vi "231215_Spectrometer_Example_2.0.vi"() -> ()   [LabVIEW 2026]
uses:
  Utils/Status_Ctrl.ctl
  Ocean Optics 2000 4000/Ocean Optics 2000 4000.lvlib
panel:
  in  "Tab Control 2":T1(tab)
  in  "Normalize?":bool
  in  "Source":u16(ring) items=["---", "Source 1", "Source 2", "Source 3"]
  out "Source graph":cluster{dbl[], dbl[]}[](graph)
  in  "SAVE":bool
  in  "Type of measurement":u16(ring)=2 items=["---", "Background noise", "Source without filter", "Source after the filter"]
  out "Source graph 2":cluster{dbl[], dbl[]}[](graph)
  out "Transmission_graph":cluster{dbl[], dbl[]}(graph)
  in  "File Path":path
  in  "File name (wo extension)":string
  in  "Type of curve to save":u16(ring)=2 items=["Save the transmission spectrum", "Save the source spectrum"]
  in  "Filter cluster":T2={"Type of filter"=enum."---", "Centered wavelength (nm)"=0.0, "Transmission band (nm)"=1.0, "Transmission (%)"=0.0} {"Transmission (%)" min=0.0 max=100.0 step=1.0; "Transmission band (nm)" min=1.0 step=1.0}
  out "Filter name":string
  out "Filter_Graph":cluster{dbl[], dbl[]}[](graph)
  out "Wavelength_Size":i32=3648
  in  "Tab Control":enum32{"Spectrometer", "Tools"}(tab)
  in  "Wavelength / Intensity limits":u16[][](array[numeric])=[[400, 0], [750, 2000]]
  in  "Intensity autoscale?":bool=TRUE
  in  "Averages":u8=1 min=1
  out "CurrentSpectrum":cluster{dbl[], dbl[]}(graph)
  out "Saturated!":bool
  in  "Status":T3=enum."Exit"
  in  "Integration time (ms)":u16=100 min=1
  out "error out":errorcluster
  # "Programmed by Sébastien Mailfert"
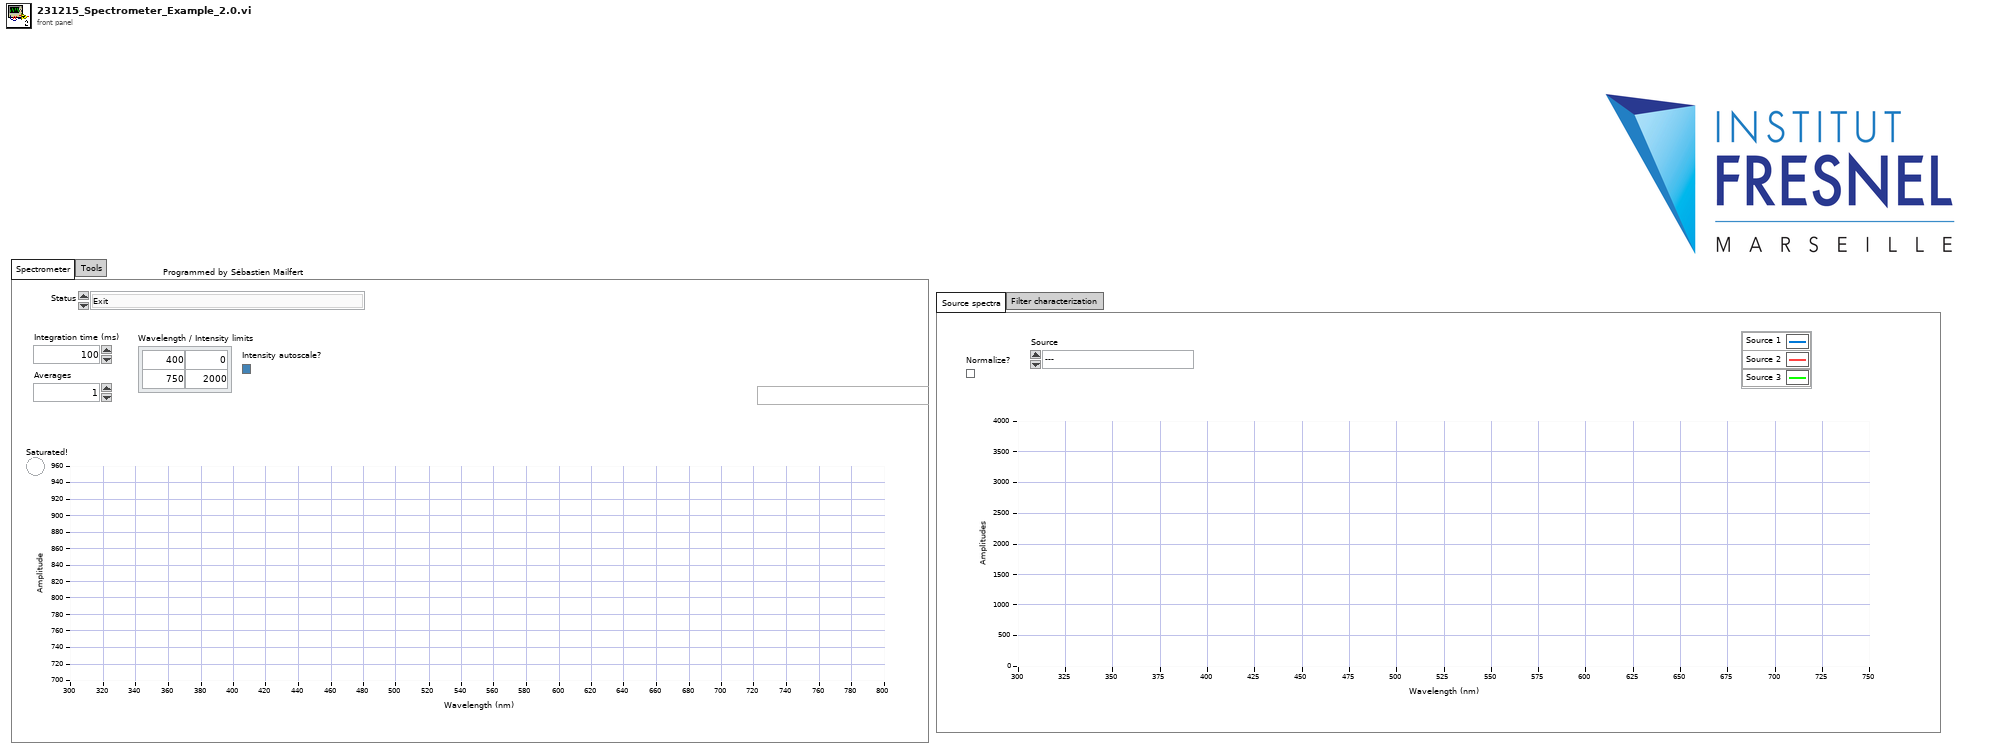
[diagram p1: front panel]
types:
  T1 = enum32{"Source spectra", "Filter characterization"}
  T2 = cluster{"Type of filter":enum16{"---", "Bandpass", "Longpass", "Shortpass"}, "Centered wavelength (nm)":dbl, "Transmission band (nm)":dbl, "Transmission (%)":dbl}
  T3 = typedef "Status_Ctrl.ctl" = enum16{"Init", "Live", "Exit"}
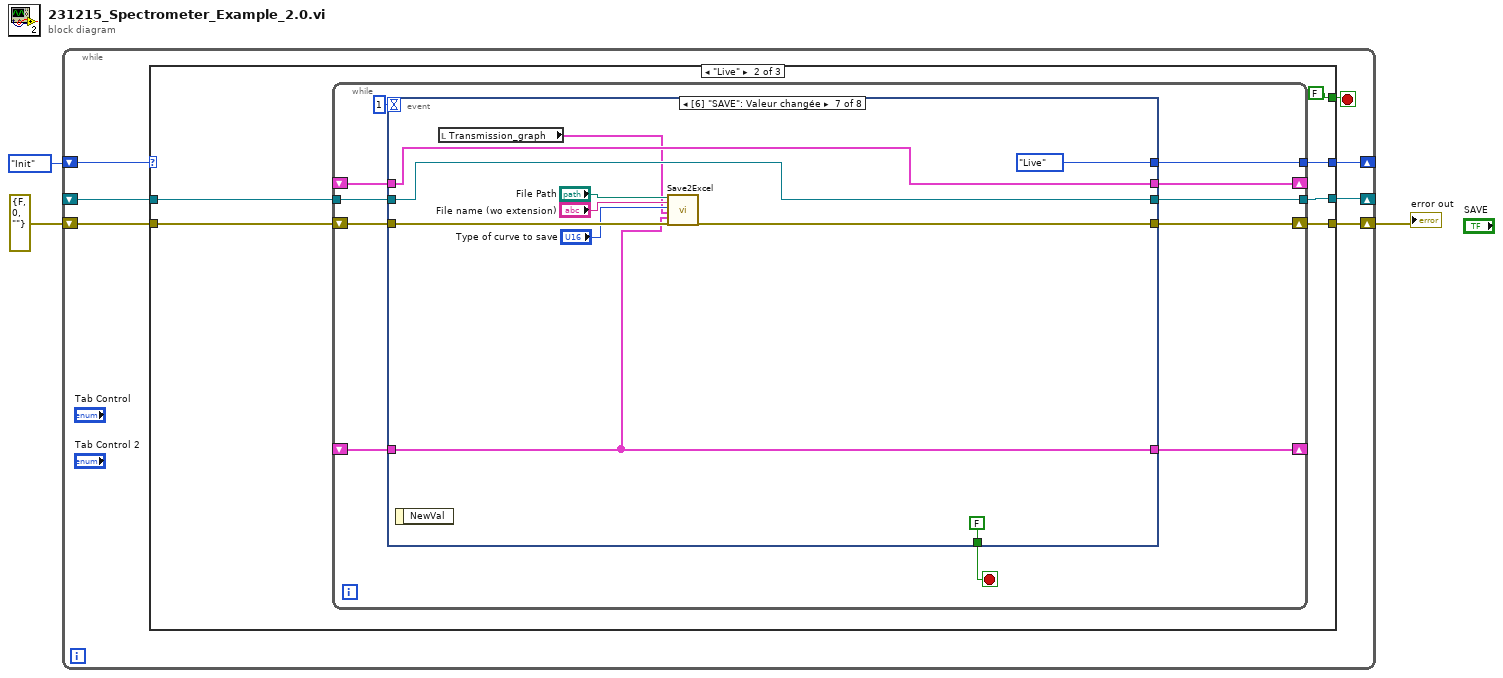
[diagram p0: block diagram]
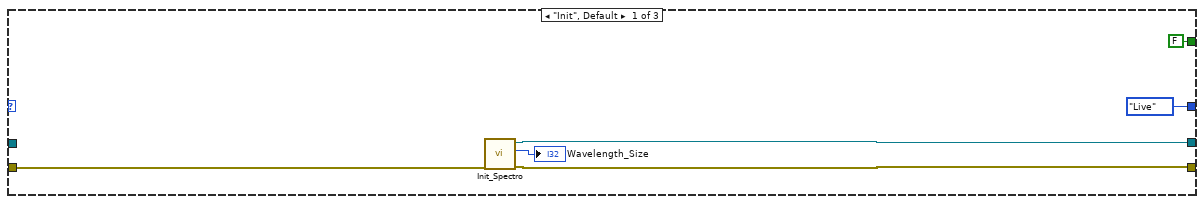
[diagram p2: hidden frame]
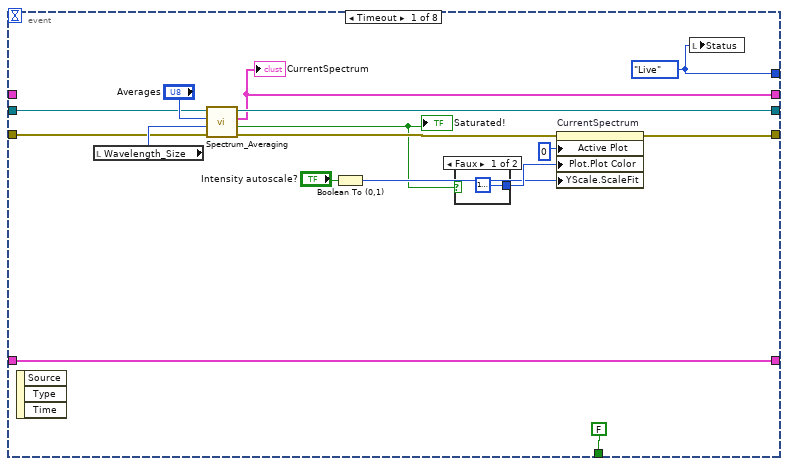
[diagram p3: hidden frame]
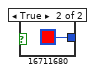
[diagram p4: hidden frame]
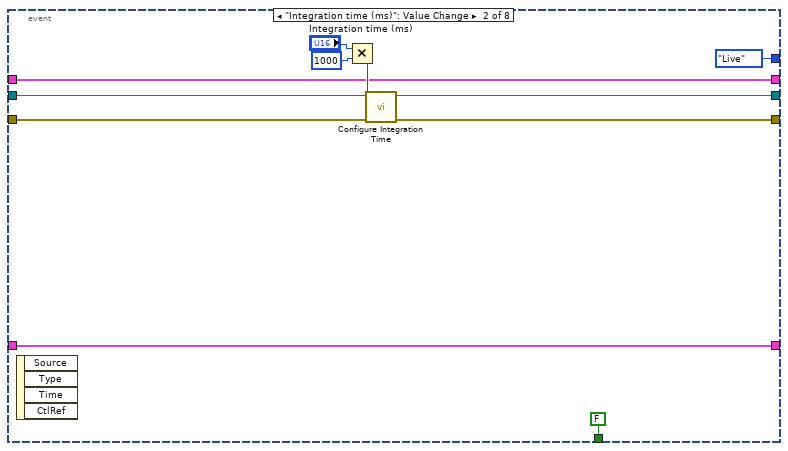
[diagram p5: hidden frame]
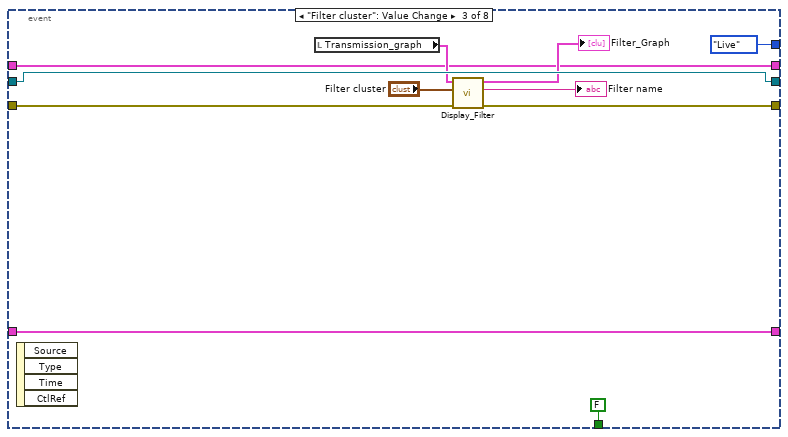
[diagram p6: hidden frame]
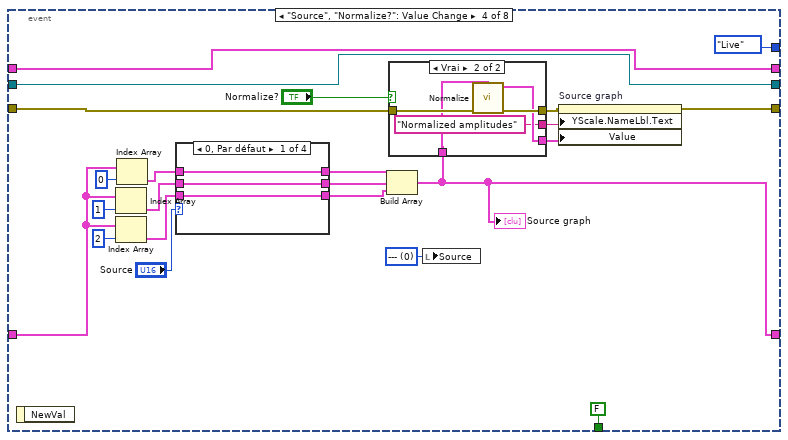
[diagram p7: hidden frame]
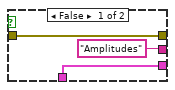
[diagram p8: hidden frame]
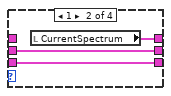
[diagram p9: hidden frame]
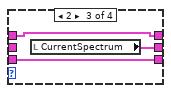
[diagram p10: hidden frame]
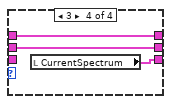
[diagram p11: hidden frame]
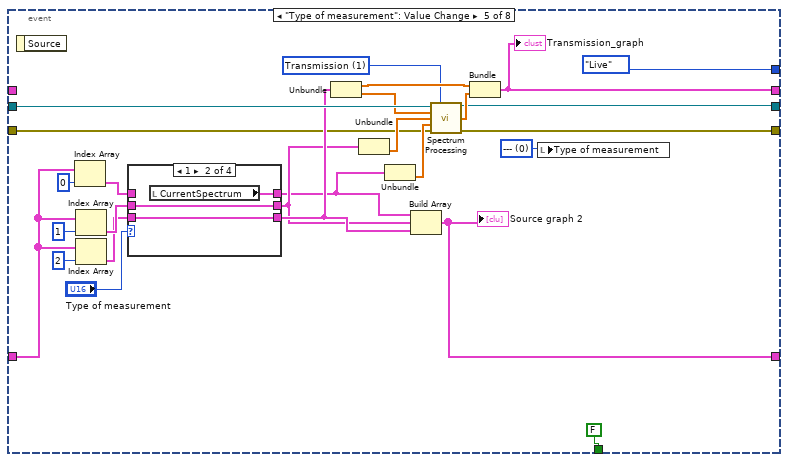
[diagram p12: hidden frame]
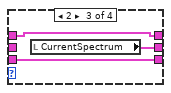
[diagram p14: hidden frame]
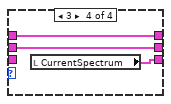
[diagram p15: hidden frame]
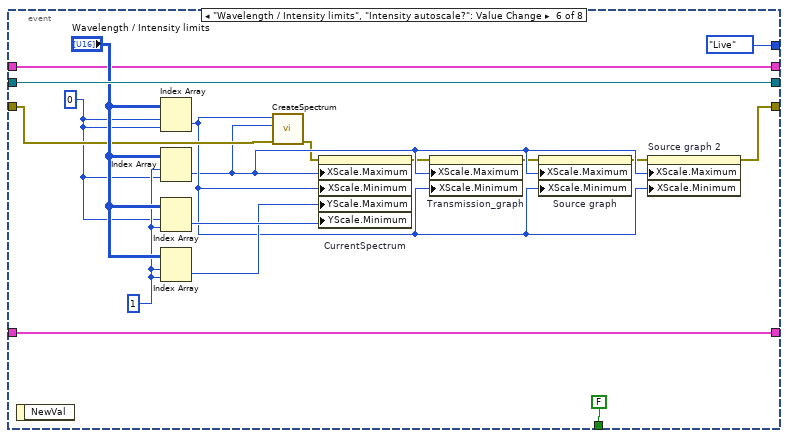
[diagram p16: hidden frame]
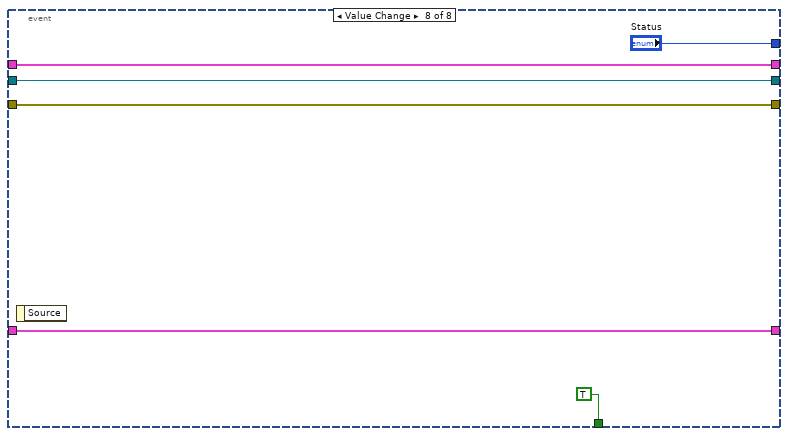
[diagram p17: hidden frame]
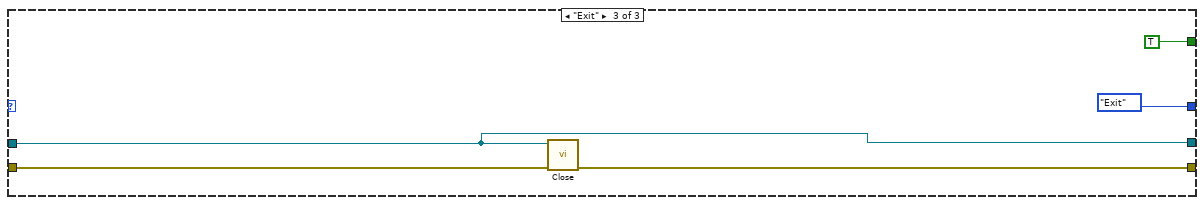
[diagram p18: hidden frame]
diagram:
  n1 = while {
    shift-right: [w9] -> _
    shift-left: Status_Ctrl."Init" ("State") -> [w8]
    shift-right: [w7] -> w1
    shift-left: errorcluster {"status"=FALSE, "code"=0, "source"=""} ("error out") -> [w6]
    shift-right: [w5] -> _
    shift-left: _ -> [w4]
    stop <- w10 stop-if-true
    n2 = case shown="\"Live\"" w8 {
      tunnel: [FALSE FALSE TRUE] -> w10
      tunnel: [Status_Ctrl."Live" ("State") w17 Status_Ctrl."Exit" ("State")] -> w9
      tunnel: [w15 w21 w191] -> w7
      tunnel: w6 -> [w14 w18 w192]
      tunnel: [w12 w20 w190] -> w5
      tunnel: w4 -> [_ w19 w190]
      frame "Init", Default {
        n3 = call "Init_Spectro.vi"("error in (no error)"=w14) -> ("error out"=w15:errorcluster, "Wavelength_Size"=→"Wavelength_Size":i32, "VISA Refnum out"=w12:refnum<visa-resource-name>)  [unwired: 8 in]
      }
      frame "Live" {
        n4 = while {
          tunnel: [w32] -> w20
          tunnel: w19 -> [w31]
          shift-right: [w33] -> w21
          shift-left: w18 -> [w30]
          tunnel: [w27] -> w17
          shift-right: [w26] -> _
          shift-left: _ -> [w25]
          shift-right: [w24] -> _
          shift-left: _ -> [w23]
          stop <- w28 stop-if-true
          n5 = event shown="[6] \"SAVE\": Valeur changée" {
            selector: _ -> [_ _ _ _ _ _ _ _]
            dyn-events: _ -> [_ _ _ _ _ _ _ _]
            timeout: 1 -> [_ _ _ _ _ _ _ _]
            tunnel: [w45 w55 w72 w78 w118 w167 w182 w189] -> w33
            tunnel: [w43 w57 w70 w96 w121 w172 w177 w188] -> w32
            tunnel: w31 -> [w35 w58 w70 w96 w131 w172 w177 w188]
            tunnel: w30 -> [w34 w59 w71 w82 w120 w168 w181 w189]
            tunnel: [FALSE FALSE FALSE FALSE FALSE FALSE FALSE TRUE] -> w28
            tunnel: [w48 Status_Ctrl."Live" ("Status") Status_Ctrl."Live" ("Status") Status_Ctrl."Live" ("State") Status_Ctrl."Live" ("State") Status_Ctrl."Live" ("State") Status_Ctrl."Live" ("Status") "Status"] -> w27
            tunnel: [w44 w52 w67 w75 w132 w162 w174 w185] -> w26
            tunnel: w25 -> [w44 w52 w67 w87 w138 w162 w174 w185]
            tunnel: [w38 w56 w63 w76 w119 w161 w176 w184] -> w24
            tunnel: w23 -> [_ w56 w63 w76 _ w161 w176 w184]
            event Timeout {
              w48 = Status_Ctrl."Live" ("State")
              n6 = event-data() -> ()  [unwired: 1 in, 3 out]
              n7 = local read "Wavelength_Size"() -> (w37:i32)
              n8 = call "Spectrum_Averaging.vi"("error in"=w34, "taille de la dimension"=w37, "Averages"="Averages", "VISA resource name in"=w35) -> ("error out"=w46:errorcluster, "Saturated?"=w36:bool, "XY Graph"=w38:cluster{dbl[], dbl[]}, "VISA resource name out"=w43:refnum<visa-resource-name>)  [unwired: 4 in]
              "CurrentSpectrum" <- w38
              "Saturated!" <- w36
              n9 = Boolean To (0,1)(Boolean="Intensity autoscale?") -> (0, 1=w40:i16)
              n10 = case shown="Faux" w36 {
                tunnel: [u32 16777224 u32 16711680] -> w42
                frame False {
                }
                frame True {
                }
              }
              n11 = property on="CurrentSpectrum" class="GraphXY (strict)"(error in=w46, "Active Plot"=u32 0, "Plot.Plot Color"=w42, "YScale.ScaleFit"=w40) -> (error out=w45:errorcluster)  [unwired: 1 in, 1 out]
              n12 = local write "Status"(w48) -> ()
            }
            event "Integration time (ms)": Value Change {
              n13 = event-data() -> ()  [unwired: 1 in, 4 out]
              n14 = Multiply(x="Integration time (ms)", y=u32 1000) -> (x*y=w61:u32)
              n15 = call "Configure Integration Time.vi"("error in (no error)"=w59, "Integration Time (6000)"=w61, "VISA resource name"=w58) -> ("error out"=w55:errorcluster, "VISA resource name out"=w57:refnum<visa-resource-name>)  [unwired: 7 in]
            }
            event "Filter cluster": Value Change {
              n16 = event-data() -> ()  [unwired: 1 in, 4 out]
              n17 = local read "Transmission_graph"() -> (w65:cluster{dbl[], dbl[]})
              n18 = call "Display_Filter.vi"("Error in"=w71, "Filter cluster"="Filter cluster", "Input data"=w65) -> ("Error out"=w72:errorcluster, "Filter name"=→"Filter name":string, "Output data"=→"Filter_Graph":cluster{dbl[], dbl[]}[])  [unwired: 6 in]
            }
            event "Source", "Normalize?": Value Change {
              w74 = u16 0 items=["---", "Xenon", "Mercury", "Laser"] ("Source")
              n19 = event-data() -> ()  [unwired: 1 in, 1 out]
              n20 = Index Array(array=w87, index=1) -> (element=w85:cluster{dbl[], dbl[]})
              n21 = Index Array(array=w87, index=2) -> (element=w84:cluster{dbl[], dbl[]})
              n22 = Index Array(array=w87, index=0) -> (element=w86:cluster{dbl[], dbl[]})
              n23 = case shown="0, Par défaut" "Source" {
                tunnel: [w106 w109 w113 w114] -> w93
                tunnel: [w107 w110 w112 w115] -> w92
                tunnel: [w105 w108 w111 w116] -> w91
                tunnel: w86 -> [w107 _ w112 w115]
                tunnel: w85 -> [w106 w109 _ w114]
                tunnel: w84 -> [w105 w108 w111 _]
                frame 0, Default {
                }
                frame 1 {
                  n24 = local read "CurrentSpectrum"() -> (w110:cluster{dbl[], dbl[]})
                }
                frame 2 {
                  n25 = local read "CurrentSpectrum"() -> (w113:cluster{dbl[], dbl[]})
                }
                frame 3 {
                  n26 = local read "CurrentSpectrum"() -> (w116:cluster{dbl[], dbl[]})
                }
              }
              n27 = Build Array(w92, w93, w91) -> (w75:cluster{dbl[], dbl[]}[])
              "Source graph" <- w75
              n28 = case shown="Vrai" "Normalize?" {
                tunnel: w82 -> [w99 w104]
                tunnel: [w99 w103] -> w79
                tunnel: [w98 w102] -> w77
                tunnel: w75 -> [w98 w101]
                tunnel: ["Amplitudes" ("Y Scale.Name Label.Text") "Normalized amplitudes" ("Y Scale.Name Label.Text")] -> w80
                frame False {
                }
                frame True {
                  n29 = call "Normalize.vi"("error in"=w104, "Source graph"=w101) -> ("error out"=w103:errorcluster, "Normalized source graph out"=w102:cluster{dbl[], dbl[]}[])  [unwired: 8 in]
                }
              }
              n30 = local write "Source"(w74) -> ()
              n31 = property on="Source graph" class="GraphXY (strict)"(error in=w79, "YScale.NameLbl.Text"=w80, "Value"=w77) -> (error out=w78:errorcluster)  [unwired: 1 in, 1 out]
            }
            event "Type of measurement": Value Change {
              w117 = u16 0 items=["---", "Background noise", "Source without filter", "Source after the filter"] ("Type of measurement")
              w122 = u16 1 items=["Absorbance", "Transmission", "Irradiance"] ("Spectral Mode (0:Absorbance)")
              n32 = event-data() -> ()  [unwired: 1 in, 1 out]
              n33 = Index Array(array=w138, index=0) -> (element=w137:cluster{dbl[], dbl[]})
              n34 = Index Array(array=w138, index=1) -> (element=w136:cluster{dbl[], dbl[]})
              n35 = Index Array(array=w138, index=2) -> (element=w135:cluster{dbl[], dbl[]})
              n36 = case shown="1" "Type of measurement" {
                tunnel: [w144 w147 w151 w152] -> w128
                tunnel: [w145 w148 w150 w153] -> w125
                tunnel: [w143 w146 w149 w154] -> w130
                tunnel: w137 -> [w145 _ w150 w153]
                tunnel: w136 -> [w144 w147 _ w152]
                tunnel: w135 -> [w143 w146 w149 _]
                frame 0, Default {
                }
                frame 1 {
                  n37 = local read "CurrentSpectrum"() -> (w148:cluster{dbl[], dbl[]})
                }
                frame 2 {
                  n38 = local read "CurrentSpectrum"() -> (w151:cluster{dbl[], dbl[]})
                }
                frame 3 {
                  n39 = local read "CurrentSpectrum"() -> (w154:cluster{dbl[], dbl[]})
                }
              }
              n40 = Unbundle(w130) -> (w124:dbl[], w129:dbl[])
              n41 = Unbundle(w128) -> (w127:dbl[])  [unwired: 1 out]
              n42 = Unbundle(w125) -> (w126:dbl[])  [unwired: 1 out]
              n43 = Build Array(w125, w128, w130) -> (w132:cluster{dbl[], dbl[]}[])
              "Source graph 2" <- w132
              n44 = call "Spectrum Processing.vi"("VISA resource name"=w131, "Spectral Mode (0:Absorbance)"=w122, "Sample Spectrum"=w129, "Reference Spectrum"=w127, "Dark Spectrum"=w126, "error in (no error)"=w120) -> ("VISA resource name out"=w121:refnum<visa-resource-name>, "Processed Spectrum"=w123:dbl[], "error out"=w118:errorcluster)  [unwired: 7 in]
              n45 = Bundle(w124, "Processed Spectrum"=w123) -> (w119:cluster{dbl[], "Processed Spectrum":dbl[]})  [unwired: 1 in]
              "Transmission_graph" <- w119
              n46 = local write "Type of measurement"(w117) -> ()
            }
            event "Wavelength / Intensity limits", "Intensity autoscale?": Value Change {
              w156 = 1 ("disabled index (row)")
              w155 = 0 ("index (row)")
              n47 = event-data() -> ()  [unwired: 1 in, 1 out]
              n48 = Index Array(array="Wavelength / Intensity limits", index (row)=w155, index (col)=w155) -> (element=w164:u16)
              n49 = Index Array(array="Wavelength / Intensity limits", index (row)=w156, index (col)=w155) -> (element=w163:u16)
              n50 = Index Array(array="Wavelength / Intensity limits", index (row)=w155, index (col)=w156) -> (element=w166:u16)
              n51 = Index Array(array="Wavelength / Intensity limits", index (row)=w156, index (col)=w156) -> (element=w165:u16)
              n52 = call "CreateSpectrum.vi"("error in (no error)"=w168, "Lambda max"=w163, "Lambda min"=w164) -> ("error out"=w159:errorcluster)  [unwired: 7 in, 1 out]
              n53 = property on="CurrentSpectrum" class="GraphXY (strict)"(error in=w159, "XScale.Maximum"=w163, "XScale.Minimum"=w164, "YScale.Maximum"=w165, "YScale.Minimum"=w166) -> (error out=w160:errorcluster)  [unwired: 1 in, 1 out]
              n54 = property on="Transmission_graph" class="GraphXY (strict)"(error in=w160, "XScale.Maximum"=w163, "XScale.Minimum"=w164) -> (error out=w158:errorcluster)  [unwired: 1 in, 1 out]
              n55 = property on="Source graph" class="GraphXY (strict)"(error in=w158, "XScale.Maximum"=w163, "XScale.Minimum"=w164) -> (error out=w157:errorcluster)  [unwired: 1 in, 1 out]
              n56 = property on="Source graph 2" class="GraphXY (strict)"(error in=w157, "XScale.Maximum"=w163, "XScale.Minimum"=w164) -> (error out=w167:errorcluster)  [unwired: 1 in, 1 out]
            }
            event "SAVE": Value Change {
              n57 = event-data() -> ()  [unwired: 1 in, 1 out]
              n58 = local read "Transmission_graph"() -> (w173:cluster{dbl[], dbl[]})
              n59 = call "Save2Excel.vi"("File Path"="File Path", "File name (wo extension)"="File name (wo extension)", "Type of curve to save"="Type of curve to save", "XY Graph"=w173, "Array"=w174, "error in (no error)"=w181) -> ("error out"=w182:errorcluster)  [unwired: 13 in]
            }
            event Value Change {
              n60 = event-data() -> ()  [unwired: 1 in, 1 out]
            }
          }
        }
      }
      frame "Exit" {
        n61 = call "Close.vi"("error in (no error)"=w192, "VISA resource name"=w190) -> ("error out"=w191:errorcluster)  [unwired: 9 in]
      }
    }
  }
  "error out" <- w1
